vi "periodicTasksRefNum.vi"() -> (1 "Refnums":T12)   [LabVIEW 2016]
uses:
  <vilib>/Rock Robotics/WPI/RobotDrive/WPI_RobotDriveDevRef.ctl
  <vilib>/Rock Robotics/WPI/MotorControl/WPI_MotorControlDeviceRef.ctl
  <vilib>/Rock Robotics/WPI/MotorControl/WPI_MotorControlType.ctl
  <vilib>/Rock Robotics/SystemInterfaces/DIO/FPGA_DIOPWMChannel.ctl
  <vilib>/Rock Robotics/WPI/PWM/WPI_PWMDeadband.ctl
  ADI MXP IMU/WPI_IMU_ADIS16448_InterruptDevRef.ctl
  ADI MXP IMU/WPI_IMU_ADIS16448_IMUDevRef.ctl
  <vilib>/Rock Robotics/SystemInterfaces/spilib/spi_bus.ctl
  <vilib>/Rock Robotics/WPI/Interrupt/WPI_InterruptRef.ctl
  <vilib>/Rock Robotics/SystemInterfaces/Interrupt/FPGA_InterruptIndex.ctl
  <vilib>/Rock Robotics/WPI/Compressor/WPI_CompressorDevRef.ctl
  <vilib>/Rock Robotics/WPI/Utilities/WPI_GetSetVariantRefNum.vi
  ADI MXP IMU/FRC_ADIS16448_IMU.lvlib
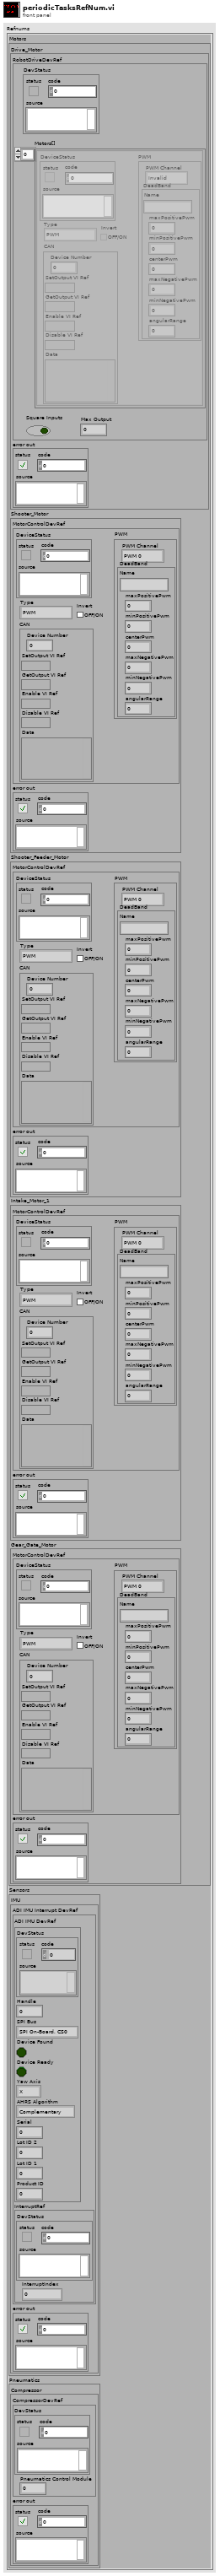
[diagram p1: front panel]
types:
  T1 = typedef "WPI_RobotDriveDevRef.ctl" = cluster{"DevStatus":errorcluster, "Motors[]":T2[], "Square Inputs":bool, "Max Output":dbl}
  T2 = typedef "WPI_MotorControlDeviceRef.ctl" = cluster{"DeviceStatus":errorcluster, "Type":T3, "PWM":cluster{"PWM Channel":T4, "DeadBand":T5}, "CAN":cluster{"Device Number":u8, "SetOutput VI Ref":variant, "GetOutput VI Ref":variant, "Enable VI Ref":variant, "Disable VI Ref":variant, "Data":variant}, "Invert":bool}
  T3 = typedef "WPI_MotorControlType.ctl" = enum16{"PWM", "CAN"}
  T4 = typedef "FPGA_DIOPWMChannel.ctl" = enum8{"PWM 0", "PWM 1", "PWM 2", "PWM 3", "PWM 4", "PWM 5", "PWM 6", "PWM 7", "PWM 8", "PWM 9", "PWM MXP 0", "PWM MXP 1", "PWM MXP 2", "PWM MXP 3", "PWM MXP 4", "PWM MXP 5", "PWM MXP 6", "PWM MXP 7", "PWM MXP 8", "PWM MXP 9", "Invalid"}
  T5 = typedef "WPI_PWMDeadband.ctl" = cluster{"Name":string, "maxPositivePwm":i32, "minPositivePwm":i32, "centerPwm":i32, "maxNegativePwm":i32, "minNegativePwm":i32, "angularRange":u16}
  T6 = typedef "FRC_ADIS16448_IMU.lvlib/WPI_IMU_ADIS16448_InterruptDevRef.ctl" = cluster{"ADI IMU DevRef":T7, "InterruptRef":T9}
  T7 = typedef "FRC_ADIS16448_IMU.lvlib/WPI_IMU_ADIS16448_IMUDevRef.ctl" = cluster{"DevStatus":errorcluster, "Handle":i32, "SPI Bus":T8, "Device Found":bool, "Device Ready":bool, "Yaw Axis":enum16{"X", "Y", "Z"}, "AHRS Algorithm":enum16{"Complementary", "Madgwick"}, "Serial":u16, "Lot ID 2":u16, "Lot ID 1":u16, "Product ID":u16}
  T8 = typedef "spi_bus.ctl" = enum16{"SPI On-Board, CS0", "SPI On-Board, CS1", "SPI On-Board, CS2", "SPI On-Board, CS3", "SPI MXP", "Invalid"}
  T9 = typedef "WPI_InterruptRef.ctl" = cluster{"DevStatus":errorcluster, "InterruptIndex":T10}
  T10 = typedef "FPGA_InterruptIndex.ctl" = enum8{"0", "1", "2", "3", "4", "5", "6", "7", "Invalid"}
  T11 = typedef "WPI_CompressorDevRef.ctl" = cluster{"DevStatus":errorcluster, "Pneumatics Control Module":u8}
  T12 = cluster{"Motors":cluster{"Drive_Motor":cluster{"RobotDriveDevRef":T1, "error out":errorcluster}, "Shooter_Motor":cluster{"MotorControlDevRef":T2, "error out":errorcluster}, "Shooter_Feeder_Motor":cluster{"MotorControlDevRef":T2, "error out":errorcluster}, "Intake_Motor_1":cluster{"MotorControlDevRef":T2, "error out":errorcluster}, "Gear_Gate_Motor":cluster{"MotorControlDevRef":T2, "error out":errorcluster}}, "Sensors":cluster{"IMU":cluster{"ADI IMU Interrupt DevRef":T6, "error out":errorcluster}}, "Pneumatics":cluster{"Compressor":cluster{"CompressorDevRef":T11, "error out":errorcluster}}}
  T13 = cluster{"Drive_Motor":cluster{"RobotDriveDevRef":T1, "error out":errorcluster}, "Shooter_Motor":cluster{"MotorControlDevRef":T2, "error out":errorcluster}, "Shooter_Feeder_Motor":cluster{"MotorControlDevRef":T2, "error out":errorcluster}, "Intake_Motor_1":cluster{"MotorControlDevRef":T2, "error out":errorcluster}, "Gear_Gate_Motor":cluster{"MotorControlDevRef":T2, "error out":errorcluster}}
  T14 = cluster{"MotorControlDevRef":T2, "error out":errorcluster}
  T15 = cluster{"Compressor":cluster{"CompressorDevRef":T11, "error out":errorcluster}}
  T16 = cluster{"CompressorDevRef":T11, "error out":errorcluster}
  T17 = cluster{"IMU":cluster{"ADI IMU Interrupt DevRef":T6, "error out":errorcluster}}
  T18 = cluster{"ADI IMU Interrupt DevRef":T6, "error out":errorcluster}
  T19 = cluster{"RobotDriveDevRef":T1, "error out":errorcluster}
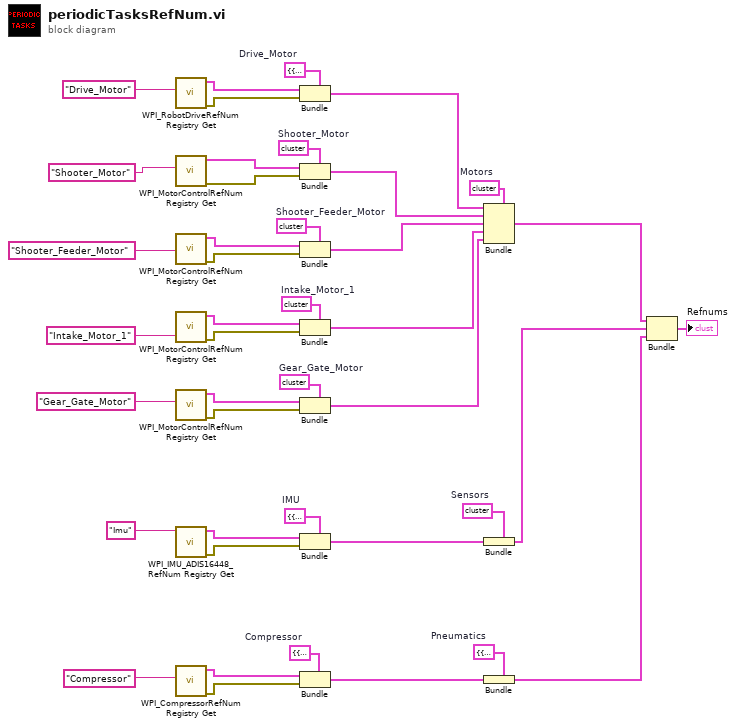
[diagram p0: block diagram]
diagram:
  w2 = T13 {"Drive_Motor"={"RobotDriveDevRef"={"DevStatus"={"status"=FALSE, "code"=0, "source"=""}, "Motors[]"=[], "Square Inputs"=FALSE, "Max Output"=0.0}, "error out"={"status"=FALSE, "code"=0, "source"=""}}, "Shooter_Motor"={"MotorControlDevRef"={"DeviceStatus"={"status"=FALSE, "code"=0, "source"=""}, "Type"=enum."PWM", "PWM"={"PWM Channel"=enum."PWM 0", "DeadBand"={"Name"="", "maxPositivePwm"=0, "minPositivePwm"=0, "centerPwm"=0, "maxNegativePwm"=0, "minNegativePwm"=0, "angularRange"=0}}, "CAN"={"Device Number"=0, "SetOutput VI Ref"=variant, "GetOutput VI Ref"=variant, "Enable VI Ref"=variant, "Disable VI Ref"=variant, "Data"=variant}, "Invert"=FALSE}, "error out"={"status"=FALSE, "code"=0, "source"=""}}, "Shooter_Feeder_Motor"={"MotorControlDevRef"={"DeviceStatus"={"status"=FALSE, "code"=0, "source"=""}, "Type"=enum."PWM", "PWM"={"PWM Channel"=enum."PWM 0", "DeadBand"={"Name"="", "maxPositivePwm"=0, "minPositivePwm"=0, "centerPwm"=0, "maxNegativePwm"=0, "minNegativePwm"=0, "angularRange"=0}}, "CAN"={"Device Number"=0, "SetOutput VI Ref"=variant, "GetOutput VI Ref"=variant, "Enable VI Ref"=variant, "Disable VI Ref"=variant, "Data"=variant}, "Invert"=FALSE}, "error out"={"status"=FALSE, "code"=0, "source"=""}}, "Intake_Motor_1"={"MotorControlDevRef"={"DeviceStatus"={"status"=FALSE, "code"=0, "source"=""}, "Type"=enum."PWM", "PWM"={"PWM Channel"=enum."PWM 0", "DeadBand"={"Name"="", "maxPositivePwm"=0, "minPositivePwm"=0, "centerPwm"=0, "maxNegativePwm"=0, "minNegativePwm"=0, "angularRange"=0}}, "CAN"={"Device Number"=0, "SetOutput VI Ref"=variant, "GetOutput VI Ref"=variant, "Enable VI Ref"=variant, "Disable VI Ref"=variant, "Data"=variant}, "Invert"=FALSE}, "error out"={"status"=FALSE, "code"=0, "source"=""}}, "Gear_Gate_Motor"={"MotorControlDevRef"={"DeviceStatus"={"status"=FALSE, "code"=0, "source"=""}, "Type"=enum."PWM", "PWM"={"PWM Channel"=enum."PWM 0", "DeadBand"={"Name"="", "maxPositivePwm"=0, "minPositivePwm"=0, "centerPwm"=0, "maxNegativePwm"=0, "minNegativePwm"=0, "angularRange"=0}}, "CAN"={"Device Number"=0, "SetOutput VI Ref"=variant, "GetOutput VI Ref"=variant, "Enable VI Ref"=variant, "Disable VI Ref"=variant, "Data"=variant}, "Invert"=FALSE}, "error out"={"status"=FALSE, "code"=0, "source"=""}}}  # Motors
  w4 = T14 {"MotorControlDevRef"={"DeviceStatus"={"status"=FALSE, "code"=0, "source"=""}, "Type"=enum."PWM", "PWM"={"PWM Channel"=enum."PWM 0", "DeadBand"={"Name"="", "maxPositivePwm"=0, "minPositivePwm"=0, "centerPwm"=0, "maxNegativePwm"=0, "minNegativePwm"=0, "angularRange"=0}}, "CAN"={"Device Number"=0, "SetOutput VI Ref"=variant, "GetOutput VI Ref"=variant, "Enable VI Ref"=variant, "Disable VI Ref"=variant, "Data"=variant}, "Invert"=FALSE}, "error out"={"status"=FALSE, "code"=0, "source"=""}}  # Gear_Gate_Motor
  w9 = T15 {"Compressor"={"CompressorDevRef"={"DevStatus"={"status"=FALSE, "code"=0, "source"=""}, "Pneumatics Control Module"=0}, "error out"={"status"=FALSE, "code"=0, "source"=""}}}  # Pneumatics
  w11 = T16 {"CompressorDevRef"={"DevStatus"={"status"=FALSE, "code"=0, "source"=""}, "Pneumatics Control Module"=0}, "error out"={"status"=FALSE, "code"=0, "source"=""}}  # Compressor
  w17 = T17 {"IMU"={"ADI IMU Interrupt DevRef"={"ADI IMU DevRef"={"DevStatus"={"status"=FALSE, "code"=0, "source"=""}, "Handle"=0, "SPI Bus"=enum."SPI On-Board, CS0", "Device Found"=FALSE, "Device Ready"=FALSE, "Yaw Axis"=enum."X", "AHRS Algorithm"=enum."Complementary", "Serial"=0, "Lot ID 2"=0, "Lot ID 1"=0, "Product ID"=0}, "InterruptRef"={"DevStatus"={"status"=FALSE, "code"=0, "source"=""}, "InterruptIndex"=enum."0"}}, "error out"={"status"=FALSE, "code"=0, "source"=""}}}  # Sensors
  w19 = T18 {"ADI IMU Interrupt DevRef"={"ADI IMU DevRef"={"DevStatus"={"status"=FALSE, "code"=0, "source"=""}, "Handle"=0, "SPI Bus"=enum."SPI On-Board, CS0", "Device Found"=FALSE, "Device Ready"=FALSE, "Yaw Axis"=enum."X", "AHRS Algorithm"=enum."Complementary", "Serial"=0, "Lot ID 2"=0, "Lot ID 1"=0, "Product ID"=0}, "InterruptRef"={"DevStatus"={"status"=FALSE, "code"=0, "source"=""}, "InterruptIndex"=enum."0"}}, "error out"={"status"=FALSE, "code"=0, "source"=""}}  # IMU
  w24 = T14 {"MotorControlDevRef"={"DeviceStatus"={"status"=FALSE, "code"=0, "source"=""}, "Type"=enum."PWM", "PWM"={"PWM Channel"=enum."PWM 0", "DeadBand"={"Name"="", "maxPositivePwm"=0, "minPositivePwm"=0, "centerPwm"=0, "maxNegativePwm"=0, "minNegativePwm"=0, "angularRange"=0}}, "CAN"={"Device Number"=0, "SetOutput VI Ref"=variant, "GetOutput VI Ref"=variant, "Enable VI Ref"=variant, "Disable VI Ref"=variant, "Data"=variant}, "Invert"=FALSE}, "error out"={"status"=FALSE, "code"=0, "source"=""}}  # Intake_Motor_1
  w34 = T14 {"MotorControlDevRef"={"DeviceStatus"={"status"=FALSE, "code"=0, "source"=""}, "Type"=enum."PWM", "PWM"={"PWM Channel"=enum."PWM 0", "DeadBand"={"Name"="", "maxPositivePwm"=0, "minPositivePwm"=0, "centerPwm"=0, "maxNegativePwm"=0, "minNegativePwm"=0, "angularRange"=0}}, "CAN"={"Device Number"=0, "SetOutput VI Ref"=variant(enum8{"Percent VBus", "Current", "Speed", "Position", "Voltage"} enum."Percent VBus"), "GetOutput VI Ref"=variant(refnum<k1> refnum), "Enable VI Ref"=variant(dbl 0.0), "Disable VI Ref"=variant(enum8{"Percent VBus", "Speed", "Position", "Slave", "Unchanged / Invalid", "Voltage Compensation", "Current", "Motion Profile"} enum."Percent VBus"), "Data"=variant}, "Invert"=FALSE}, "error out"={"status"=FALSE, "code"=0, "source"=""}}  # Shooter_Feeder_Motor
  w35 = T14 {"MotorControlDevRef"={"DeviceStatus"={"status"=FALSE, "code"=0, "source"=""}, "Type"=enum."PWM", "PWM"={"PWM Channel"=enum."PWM 0", "DeadBand"={"Name"="", "maxPositivePwm"=0, "minPositivePwm"=0, "centerPwm"=0, "maxNegativePwm"=0, "minNegativePwm"=0, "angularRange"=0}}, "CAN"={"Device Number"=0, "SetOutput VI Ref"=variant(enum8{"Percent VBus", "Current", "Speed", "Position", "Voltage"} enum."Percent VBus"), "GetOutput VI Ref"=variant(refnum<k1> refnum), "Enable VI Ref"=variant(dbl 0.0), "Disable VI Ref"=variant(enum8{"Percent VBus", "Speed", "Position", "Slave", "Unchanged / Invalid", "Voltage Compensation", "Current", "Motion Profile"} enum."Percent VBus"), "Data"=variant}, "Invert"=FALSE}, "error out"={"status"=FALSE, "code"=0, "source"=""}}  # Shooter_Motor
  w39 = T19 {"RobotDriveDevRef"={"DevStatus"={"status"=FALSE, "code"=0, "source"=""}, "Motors[]"=[], "Square Inputs"=FALSE, "Max Output"=0.0}, "error out"={"status"=FALSE, "code"=0, "source"=""}}  # Drive_Motor
  n1 = call <vilib>:"WPI_RobotDriveRefNum Registry Get.vi"("refnum name"="Drive_Motor") -> ("error out"=w40:errorcluster, "RobotDriveDevRef"=w41:T1)  [unwired: 9 in]
  n2 = call <vilib>:"WPI_MotorControlRefNum Registry Get.vi"("refnum name"="Shooter_Motor") -> ("error out"=w29:errorcluster, "MotorControlDevRef"=w30:T2)  [unwired: 9 in]
  n3 = call <vilib>:"WPI_MotorControlRefNum Registry Get.vi"("refnum name"="Shooter_Feeder_Motor") -> ("error out"=w27:errorcluster, "MotorControlDevRef"=w28:T2)  [unwired: 9 in]
  n4 = call <vilib>:"WPI_MotorControlRefNum Registry Get.vi"("refnum name"="Intake_Motor_1") -> ("error out"=w25:errorcluster, "MotorControlDevRef"=w26:T2)  [unwired: 9 in]
  n5 = call <vilib>:"WPI_MotorControlRefNum Registry Get.vi"("refnum name"="Gear_Gate_Motor") -> ("error out"=w6:errorcluster, "MotorControlDevRef"=w5:T2)  [unwired: 9 in]
  n6 = call "WPI_IMU_ADIS16448_RefNum Registry Get.vi"("refnum name"="Imu") -> ("error out"=w20:errorcluster, "ADI IMU Interrupt DevRef"=w21:T6)  [unwired: 9 in]
  n7 = call <vilib>:"WPI_CompressorRefNum Registry Get.vi"("refnum name"="Compressor") -> ("error out"=w12:errorcluster, "CompressorDevRef"=w13:T11)  [unwired: 9 in]
  n8 = Bundle(cluster=w39, "RobotDriveDevRef"=w41, "error out"=w40) -> (w38:T19)
  n9 = Bundle(cluster=w35, "MotorControlDevRef"=w30, "error out"=w29) -> (w37:T14)
  n10 = Bundle(cluster=w34, "MotorControlDevRef"=w28, "error out"=w27) -> (w36:T14)
  n11 = Bundle(cluster=w24, "MotorControlDevRef"=w26, "error out"=w25) -> (w23:T14)
  n12 = Bundle(cluster=w4, "MotorControlDevRef"=w5, "error out"=w6) -> (w3:T14)
  n13 = Bundle(cluster=w19, "ADI IMU Interrupt DevRef"=w21, "error out"=w20) -> (w18:T18)
  n14 = Bundle(cluster=w11, "CompressorDevRef"=w13, "error out"=w12) -> (w10:T16)
  n15 = Bundle(cluster=w2, "Drive_Motor"=w38, "Shooter_Motor"=w37, "Shooter_Feeder_Motor"=w36, "Intake_Motor_1"=w23, "Gear_Gate_Motor"=w3) -> (w16:T13)
  n16 = Bundle(cluster=w17, "IMU"=w18) -> (w15:T17)
  n17 = Bundle(cluster=w9, "Compressor"=w10) -> (w8:T15)
  n18 = Bundle("Motors"=w16, "Sensors"=w15, "Pneumatics"=w8) -> (→"Refnums":T12)  [unwired: 1 in]
